vi "PID.vi"(6 "stop":bool, 7 "Angulo Deseado 2":dbl step=100.0, 8 "Reset Counter 2":bool, 9 "Reset Counter":bool, 10 "Angulo Deseado 1":dbl) -> (2 "Pulsos 2":i32, 3 "Pulsos 1":i32)   [LabVIEW 2019]
uses:
  <vilib>/Platform/TimedLoop/XDataNode/timing_clust.ctl
  <vilib>/Platform/TimedLoop/XDataNode/nitl_modes.ctl
  <vilib>/Platform/TimedLoop/XDataNode/wakeup.ctl
  <vilib>/myRIO/Common/Instrument Driver Framework/myRIO v1.0/Encoder/typedefs/Encoder Signal Mode.ctl
  <vilib>/myRIO/Common/Instrument Driver Framework/myRIO v1.0/UART/vis/myRIO v1.0 Close UART.vi
  <vilib>/Utility/error.llb/Error Cluster From Error Code.vi
  <vilib>/myRIO/Common/Instrument Driver Framework/myRIO v1.0/Encoder/vis/myRIO v1.0 Read Encoder.vi
  <vilib>/myRIO/Common/Instrument Driver Framework/myRIO v1.0/PWM/vis/myRIO v1.0 Write PWM.vi
  <vilib>/myRIO/Common/Instrument Driver Framework/myRIO v1.0/DIO/vis/myRIO v1.0 Write DIO.vi
  <vilib>/myRIO/Common/Instrument Driver Framework/Utilities/vis/FPGA Ref Manager.vi
  <vilib>/myRIO/Common/Instrument Driver Framework/myRIO v1.0/myRIO v1.0 Reset FPGA.vi
  <vilib>/myRIO/Common/Instrument Driver Framework/myRIO v1.0/IRQ/vis/myRIO v1.0 IRQ Info FGV.vi
  <vilib>/myRIO/Common/Instrument Driver Framework/myRIO v1.0/IRQ/vis/myRIO v1.0 Timer IRQ Info FGV.vi
  <vilib>/myRIO/Common/Instrument Driver Framework/myRIO v1.0/IRQ/vis/myRIO v1.0 ISR Agent.vi
  <vilib>/myRIO/Instrument Drivers/Utilities/vis/Reset Index.vi
  <vilib>/myRIO/Common/Instrument Driver Framework/myRIO v1.0/Resource Manager/vis/myRIO v1.0 Block Write Resource Manager.vi
  <vilib>/platform/TimedLoop/XDataNode/XDataNode.xnode
  <vilib>/Platform/TimedLoop/XDataNode/XDNodeRunTimeDep.lvlib
  <vilib>/myRIO/Instrument Drivers/Onboard IO/Encoder/Encoder.lvlib
  <vilib>/myRIO/Instrument Drivers/Onboard IO/PWM/PWM.lvlib
  <vilib>/myRIO/Instrument Drivers/Onboard IO/DIO/DIO.lvlib
  <vilib>/myRIO/Instrument Drivers/Utilities/Utilities.lvlib
panel:
  out "Numeric":dbl
  out "Td2":dbl
  out "Ti2":dbl
  out "Kp2":dbl
  out "Td1":dbl
  out "Ti1":dbl
  out "Kp1":dbl
  in  "error 2":dbl
  in  "error":dbl
  out "Waveform Chart":dbl(graph)
  in  "Wc filtro digital 2":dbl
  in  "Wc filtro digital":dbl
  out "Tiempo de muestreo":dbl
  out "?":cluster{dbl, dbl}(graph)
  out "?":cluster{dbl, dbl}(graph)
  out "Angulo Motor 1":dbl
  out "Angulo Motor 2":dbl
  out "Velocidad Motor1":dbl caption="rad/s"
  out "Velocidad Motor2":dbl caption="rad/s"
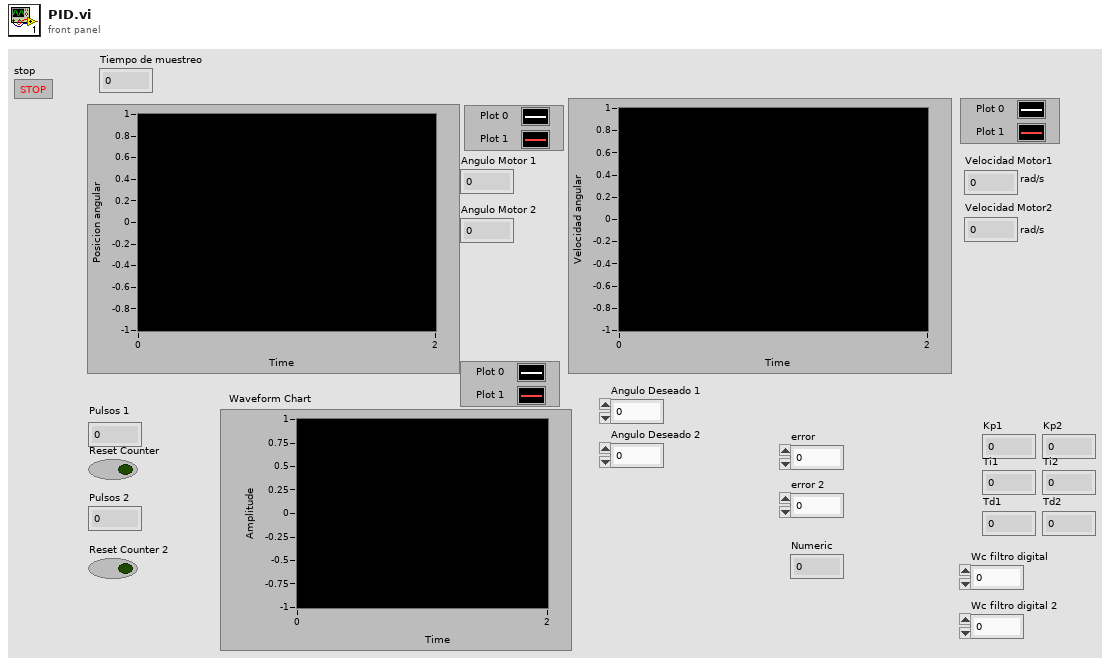
[diagram p1: front panel]
types:
  T1 = typedef "XDNodeRunTimeDep.lvlib/timing_clust.ctl" = cluster{"Expected End [f-1]":u64, "Actual End [f-1]":u64, "Finished Late? [f-1]":bool, "Expected End [i-1]":u64, "Actual End [i-1]":u64, "Finished Late? [i-1]":bool, "Expected Start [i]":u64, "Actual Start [i]":u64, "Expected Start [f]":u64, "Actual Start [f]":u64, "Source Name":string, "Structure Name":string, "Period":i64, "Deadline":i64, "Offset":i64, "Start":i64, "Priority":i32, "Timeout":i32, "Mode":T2, "Wakeup Reason":T3, "Error":errorcluster, "Source Type":string, "Secondary Source Type":string, "Global End Time":u64, "Global Start Time":u64, "Frame Duration":u64, "Iteration Duration":u64, "Assigned CPU":i32, "I/O Scan Engine Mode":u32}
  T2 = typedef "XDNodeRunTimeDep.lvlib/nitl_modes.ctl" = enum32{"No Change", "Process missed periods, maintain original phase", "Discard missed periods, maintain original phase", "Process missed periods, ignore original phase", "Discard missed periods, ignore original phase"}
  T3 = typedef "XDNodeRunTimeDep.lvlib/wakeup.ctl" = enum32{"Normal", "Aborted", "Asynchronous wakeup", "Timing source error", "Timed loop error", "Timeout"}
  T4 = typedef "PWM.lvlib/PWM Reference.ctl" = cluster{"myRIO Reference":T5, "PWM Channels Enum":T9, "PWM Configuration":T10}
  T5 = typedef "myRIO Generic Hardware Reference.ctl" = cluster{"myRIO Model":T6, "myRIO Hardware Reference":T7}
  T6 = typedef "Hardware Version Enum.ctl" = enum16{"Unknown", "myRIO-1900", "myRIO-1950", "roboRIO", "NI ELVIS RIO CM", "ELVIS III"}
  T7 = typedef "myRIO v1.0 Reference.ctl" = cluster{"Generic FPGA Reference":T8, "Allow multiple opens":bool}
  T8 = typedef "Generic FPGA Reference.ctl" = refnum<k20>
  T9 = typedef "PWM Channels Enum.ctl" = enum16{"Not Connected", "C/PWM0", "C/PWM1", "A/PWM0", "A/PWM1", "A/PWM2", "A/PWM3", "A/PWM4", "A/PWM5", "A/PWM6", "A/PWM7", "A/PWM8", "A/PWM9", "A/PWM10", "A/PWM11", "A/PWM12", "A/PWM13", "A/PWM14", "A/PWM15", "A/PWM16", "A/PWM17", "A/PWM18", "A/PWM19", "B/PWM0", "B/PWM1", "B/PWM2", "B/PWM3", "B/PWM4", "B/PWM5", "B/PWM6", "B/PWM7", "B/PWM8", "B/PWM9", "B/PWM10", "B/PWM11", "B/PWM12", "B/PWM13", "B/PWM14", "B/PWM15", "B/PWM16", "B/PWM17", "B/PWM18", "B/PWM19", "PWM/PWM0", "PWM/PWM1", "PWM/PWM2", "PWM/PWM3", "PWM/PWM4", "PWM/PWM5", "PWM/PWM6", "PWM/PWM7", "PWM/PWM8", "PWM/PWM9"}
  T10 = typedef "PWM.lvlib/PWM Configuration.ctl" = cluster{"Frequency":dbl, "Duty Cycle":dbl}
  T11 = typedef "DIO.lvlib/DIO Reference.ctl" = cluster{"myRIO Reference":T5, "DIO Channels List":T12}
  T12 = typedef "DIO Channels List.ctl" = T13[]
  T13 = typedef "DIO Channels Enum.ctl" = enum16{"Not Connected", "C/DIO0", "C/DIO1", "C/DIO2", "C/DIO3", "C/DIO4", "C/DIO5", "C/DIO6", "C/DIO7", "A/DIO0", "A/DIO1", "A/DIO2", "A/DIO3", "A/DIO4", "A/DIO5", "A/DIO6", "A/DIO7", "A/DIO8", "A/DIO9", "A/DIO10", "A/DIO11", "A/DIO12", "A/DIO13", "A/DIO14", "A/DIO15", "A/DIO16", "A/DIO17", "A/DIO18", "A/DIO19", "B/DIO0", "B/DIO1", "B/DIO2", "B/DIO3", "B/DIO4", "B/DIO5", "B/DIO6", "B/DIO7", "B/DIO8", "B/DIO9", "B/DIO10", "B/DIO11", "B/DIO12", "B/DIO13", "B/DIO14", "B/DIO15", "B/DIO16", "B/DIO17", "B/DIO18", "B/DIO19", "LED0", "LED1", "LED2", "LED3", "Button0", "DIO/DIO0", "DIO/DIO1", "DIO/DIO2", "DIO/DIO3", "DIO/DIO4", "DIO/DIO5", "DIO/DIO6", "DIO/DIO7", "DIO/DIO8", "DIO/DIO9", "SPI/CS0", "SPI/CS1", "SPI/CS2", "SPI/CS3", "LED RADIO (Green)", "LED RADIO (Red)", "LED COMM (Green)", "LED COMM (Red)", "LED MODE (Green)", "LED MODE (Red)"}
  T14 = typedef "Encoder Signal Mode.ctl" = enum16{"Quadrature phase signal", "Step and direction signal"}
  T15 = typedef "Encoder.lvlib/Encoder Reference.ctl" = cluster{"myRIO Reference":T5, "Encoder Channels Enum":T16}
  T16 = typedef "Encoder Channels Enum.ctl" = enum16{"Not Connected", "C/ENC0", "C/ENC1", "A/ENC", "A/ENC0", "A/ENC1", "A/ENC2", "A/ENC3", "A/ENC4", "A/ENC5", "A/ENC6", "A/ENC7", "A/ENC8", "A/ENC9", "B/ENC", "B/ENC0", "B/ENC1", "B/ENC2", "B/ENC3", "B/ENC4", "B/ENC5", "B/ENC6", "B/ENC7", "B/ENC8", "B/ENC9", "DIO/ENC0", "DIO/ENC1", "DIO/ENC2", "DIO/ENC3", "DIO/ENC4"}
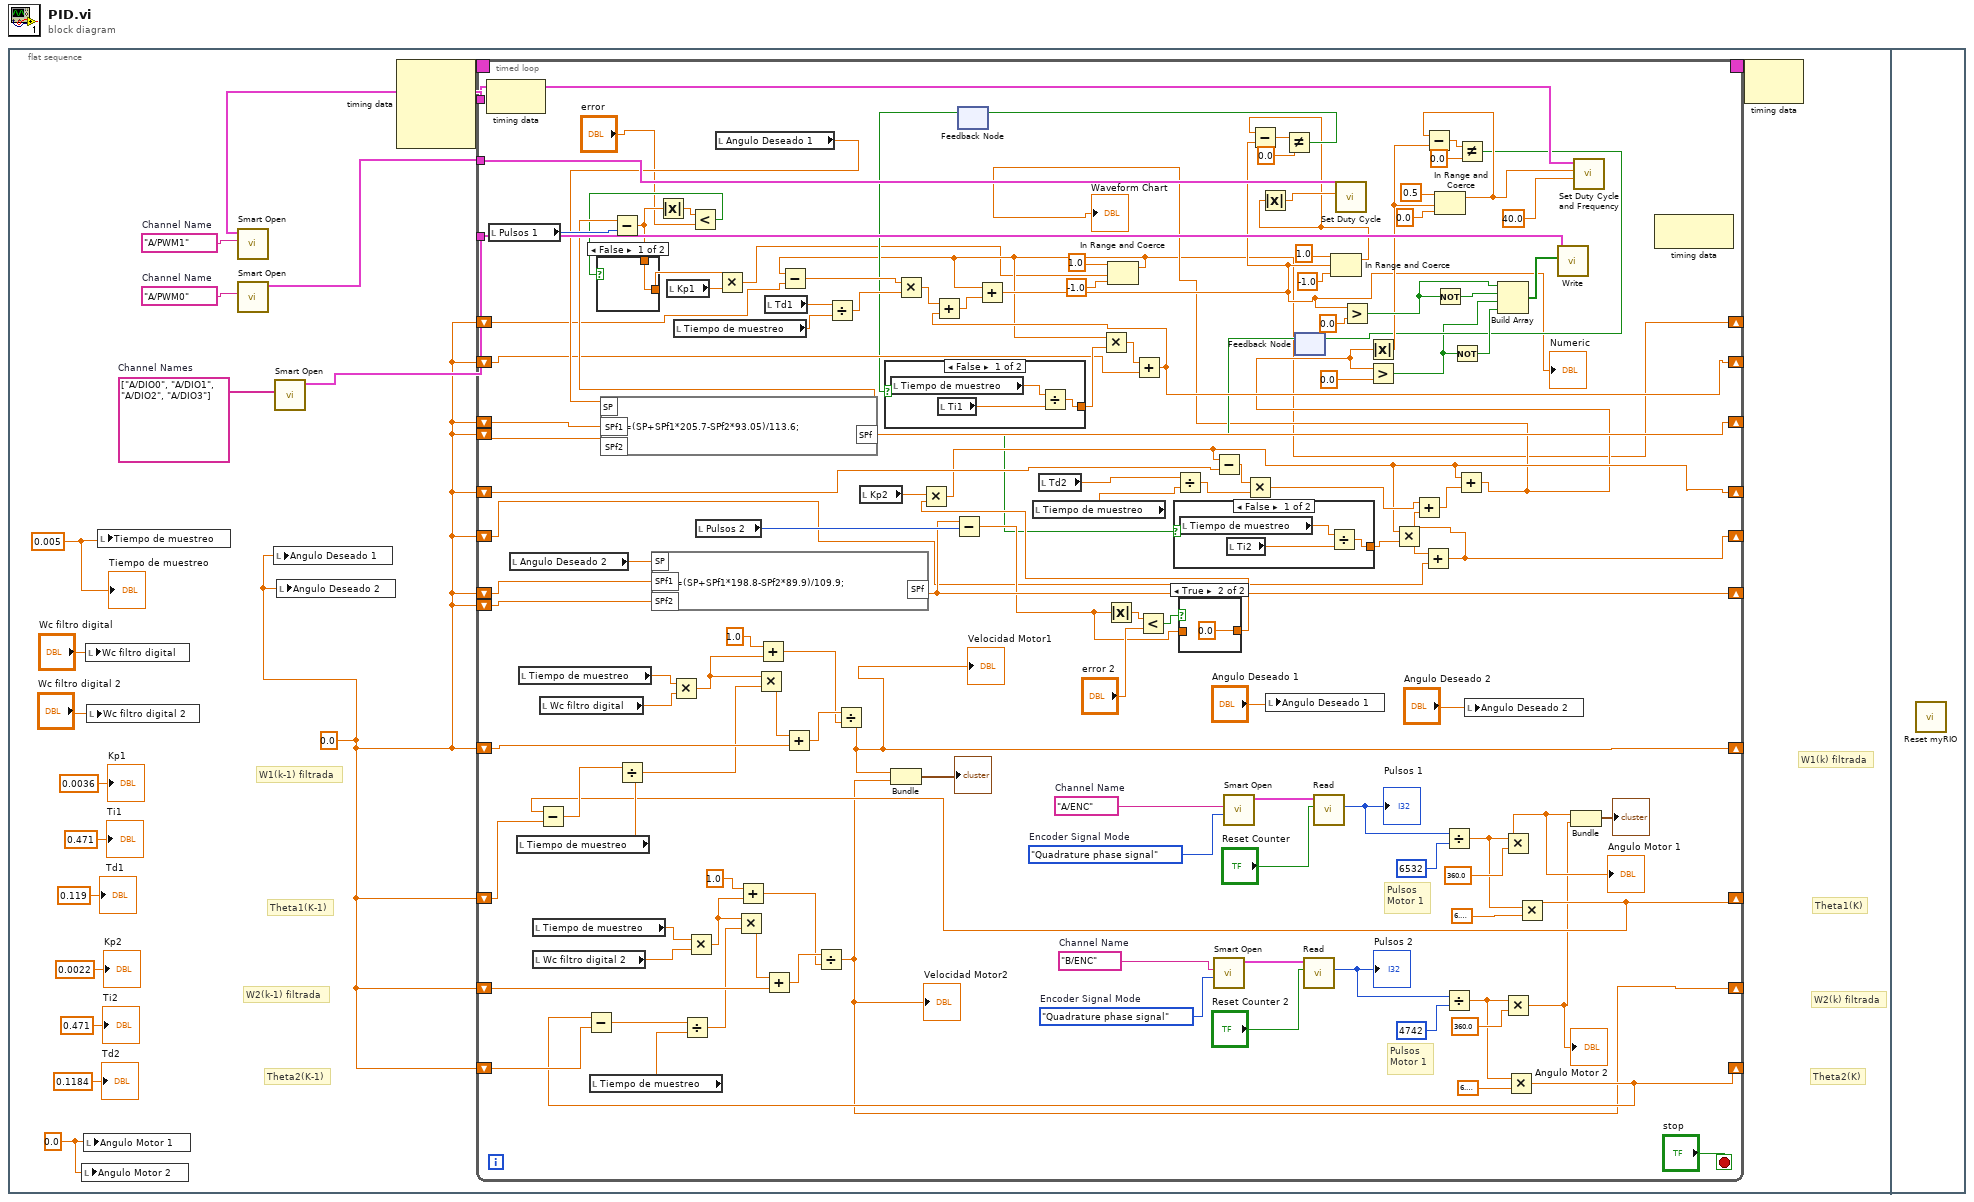
[diagram p0: block diagram]
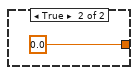
[diagram p2: hidden frame]
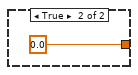
[diagram p3: hidden frame]
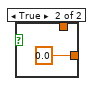
[diagram p5: hidden frame]
diagram:
  n1 = flat-sequence {
    frame #0 {
      w9 = tag "A/PWM1"  # Channel Name
      w1 = 0.0
      w10 = 0.0 ("Angulo Motor 1")
      w12 = tag[] ["A/DIO0", "A/DIO1", "A/DIO2", "A/DIO3"]  # Channel Names
      w15 = 0.005 ("Tiempo de muestreo")
      w16 = tag "A/PWM0"  # Channel Name
      # "W1(k-1) filtrada"
      # "W1(k) filtrada"
      # "Theta1(K-1)"
      # "Theta2(K-1)"
      # "W2(k-1) filtrada"
      # "Theta1(K)"
      # "Theta2(K)"
      # "W2(k) filtrada"
      n2 = local write "Angulo Motor 2"(w10) -> ()
      n3 = local write "Angulo Motor 1"(w10) -> ()
      n4 = local write "Wc filtro digital"("Wc filtro digital") -> ()
      n5 = local write "Wc filtro digital 2"("Wc filtro digital 2") -> ()
      n6 = local write "Tiempo de muestreo"(w15) -> ()
      n7 = call <vilib>:"Smart Open.vi"("Channel Name"=w9) -> ("PWM Ref Out"=w8:T4)  [unwired: 9 in, 1 out]
      n8 = call <vilib>:"Smart Open.vi"("Channel Name"=w16) -> ("PWM Ref Out"=w17:T4)  [unwired: 9 in, 1 out]
      n9 = local write "Angulo Deseado 1"(w1) -> ()
      n10 = call <vilib>:"Smart Open.vi"("Channel Names"=w12) -> ("DIO Ref Out"=w11:T11)  [unwired: 9 in, 1 out]
      n11 = local write "Angulo Deseado 2"(w1) -> ()
      n12 = node-c288() -> (w19:T1)  [unwired: 4 in]
      n13 = timed-loop {
        timing: w19 -> [_]
        timing-out: [_] -> w18
        shift-right: [w129] -> _
        shift-left: w1 -> [w130]
        shift-right: [w104] -> _
        shift-left: w1 -> [w131]
        tunnel: w17 -> [w123]
        shift-right: [w100] -> _
        shift-left: w1 -> [w118]
        shift-right: [w99] -> _
        shift-left: w1 -> [w107]
        tunnel: w11 -> [w105]
        tunnel: w8 -> [w69]
        shift-right: [w40] -> _
        shift-left: w1 -> [w41]
        shift-right: [w37] -> _
        shift-left: w1 -> [w45]
        shift-right: [w83] -> _
        shift-left: w1 -> [w85]
        shift-left: w1 -> [w84]
        shift-right: [w78] -> _
        shift-left: w1 -> [w81]
        shift-left: w1 -> [w80]
        shift-right: [w22] -> _
        shift-left: w1 -> [w62]
        shift-right: [w58] -> _
        shift-left: w1 -> [w59]
        stop <- "stop" stop-if-true
        w145 = Encoder_Signal_Mode."Quadrature phase signal"  # Encoder Signal Mode
        w146 = tag "B/ENC"  # Channel Name
        w149 = Encoder_Signal_Mode."Quadrature phase signal"  # Encoder Signal Mode
        w150 = tag "A/ENC"  # Channel Name
        # "Pulsos\nMotor 1"
        # "Pulsos\nMotor 1"
        n14 = node-c288() -> ()  [unwired: 1 in, 1 out]
        n15 = local read "Pulsos 1"() -> (w79:i32)
        n16 = local read "Angulo Deseado 2"() -> (w86:dbl)
        n17 = local read "Tiempo de muestreo"() -> (w125:dbl)
        n18 = local read "Tiempo de muestreo"() -> (w121:dbl)
        n19 = local read "Tiempo de muestreo"() -> (w120:dbl)
        n20 = local read "Wc filtro digital 2"() -> (w119:dbl)
        n21 = local read "Wc filtro digital"() -> (w122:dbl)
        n22 = local read "Tiempo de muestreo"() -> (w124:dbl)
        n23 = formula code="SPf=(SP+SPf1*198.8-SPf2*89.9)/109.9;"("SPf1"=w85, "SPf2"=w84, "SP"=w86) -> ("SPf"=w83:dbl)
        n24 = local read "Kp1"() -> (w68:dbl)
        n25 = Multiply(x=w121, y=w122) -> (x*y=w108:dbl)
        n26 = local read "Tiempo de muestreo"() -> (w66:dbl)
        n27 = Multiply(x=w120, y=w119) -> (x*y=w115:dbl)
        n28 = local read "Pulsos 2"() -> (w87:i32)
        n29 = local read "Angulo Deseado 1"() -> (w73:dbl)
        n30 = formula code="SPf=(SP+SPf1*205.7-SPf2*93.05)/113.6;"("SPf1"=w81, "SPf2"=w80, "SP"=w73) -> ("SPf"=w78:dbl)
        n31 = Subtract(x=w78, y=w79) -> (x-y=w74:dbl)
        n32 = Absolute Value(x=w74) -> (abs(x)=w76:dbl)
        n33 = Less?(x=w76, y="error") -> (x < y?=w75:bool)
        n34 = case shown="False" w75 {
          tunnel: [w161 0.0] -> w67
          tunnel: w74 -> [w161 _]
          frame False {
          }
          frame True {
          }
        }
        n35 = Multiply(x=w67, y=w68) -> (x*y=w21:dbl)
        n36 = Add(x=1.0, y=w115) -> (x+y=w112:dbl)
        n37 = Add(x=1.0, y=w108) -> (x+y=w109:dbl)
        n38 = local read "Td1"() -> (w65:dbl)
        n39 = Divide(x=w65, y=w66) -> (x/y=w64:dbl)
        n40 = local read "Kp2"() -> (w48:dbl)
        n41 = Subtract(x=w83, y=w87) -> (x-y=w47:dbl)
        n42 = feedback #1() -> (w52:bool)  [unwired: 1 in]
        n43 = case shown="False" w52 {
          tunnel: [w155 0.0] -> w61
          frame False {
            n44 = local read "Tiempo de muestreo"() -> (w156:dbl)
            n45 = local read "Ti1"() -> (w157:dbl)
            n46 = Divide(x=w156, y=w157) -> (x/y=w155:dbl)
          }
          frame True {
          }
        }
        n47 = local read "Tiempo de muestreo"() -> (w51:dbl)
        n48 = local read "Td2"() -> (w50:dbl)
        n49 = Absolute Value(x=w47) -> (abs(x)=w71:dbl)
        n50 = In Range and Coerce(upper limit=1.0, x=w21, lower limit=-1.0) -> (coerced(x)=w22:dbl)  [unwired: 1 out]
        n51 = Subtract(x=w22, y=w62) -> (x-y=w63:dbl)
        n52 = Multiply(x=w63, y=w64) -> (x*y=w57:dbl)
        n53 = Multiply(x=w22, y=w61) -> (x*y=w60:dbl)
        n54 = Add(x=w60, y=w59) -> (x+y=w58:dbl)
        n55 = Add(x=w57, y=w58) -> (x+y=w56:dbl)
        n56 = Add(x=w22, y=w56) -> (x+y=w26:dbl)
        "Numeric" <- w26
        n57 = Less?(x=w71, y="error 2") -> (x < y?=w30:bool)
        n58 = Divide(x=w50, y=w51) -> (x/y=w49:dbl)
        n59 = case shown="True" w30 {
          tunnel: [w159 0.0] -> w46
          tunnel: w47 -> [w159 _]
          frame False {
          }
          frame True {
          }
        }
        n60 = Multiply(x=w48, y=w46) -> (x*y=w37:dbl)
        n61 = Subtract(x=w37, y=w45) -> (x-y=w44:dbl)
        n62 = call <vilib>:"Smart Open.vi"("Encoder Signal Mode"=w145, "Channel Name"=w146) -> ("Encoder Ref Out"=w143:T15)  [unwired: 8 in, 1 out]
        n63 = call <vilib>:"Smart Open.vi"("Encoder Signal Mode"=w149, "Channel Name"=w150) -> ("Encoder Ref Out"=w147:T15)  [unwired: 8 in, 1 out]
        n64 = Multiply(x=w44, y=w49) -> (x*y=w39:dbl)
        n65 = local write "Angulo Deseado 1"("Angulo Deseado 1") -> ()
        n66 = feedback #2() -> (w31:bool)  [unwired: 1 in]
        n67 = case shown="False" w31 {
          tunnel: [w151 0.0] -> w43
          frame False {
            n68 = local read "Tiempo de muestreo"() -> (w152:dbl)
            n69 = local read "Ti2"() -> (w153:dbl)
            n70 = Divide(x=w152, y=w153) -> (x/y=w151:dbl)
          }
          frame True {
          }
        }
        n71 = call <vilib>:"Read.vi"("Reset Counter"="Reset Counter 2", "Encoder Ref In"=w143) -> ("Counter Value"=w136:i32)  [unwired: 5 in, 4 out]
        "Pulsos 2" <- w136
        n72 = call <vilib>:"Read.vi"("Reset Counter"="Reset Counter", "Encoder Ref In"=w147) -> ("Counter Value"=w142:i32)  [unwired: 5 in, 4 out]
        "Pulsos 1" <- w142
        n73 = In Range and Coerce(upper limit=1.0, x=w26, lower limit=-1.0) -> (coerced(x)=w27:dbl)  [unwired: 1 out]
        n74 = Subtract(x=w27, y=w26) -> (x-y=w55:dbl)
        n75 = Absolute Value(x=w27) -> (abs(x)=w28:dbl)
        n76 = Not Equal?(x=w55, y=0.0) -> (x != y?=w53:bool)
        n77 = feedback-in #1(w53) -> ()
        n78 = call <vilib>:"Set Duty Cycle.vi"("Duty Cycle"=w28, "PWM Ref In"=w123) -> ()  [unwired: 7 in, 2 out]
        n79 = Greater?(x=w26, y=0.0) -> (0:w82:bool)
        n80 = Multiply(x=w37, y=w43) -> (x*y=w42:dbl)
        n81 = Add(x=w42, y=w41) -> (x+y=w40:dbl)
        n82 = Add(x=w39, y=w40) -> (x+y=w38:dbl)
        n83 = Not(x=w82) -> (.not. x?=w97:bool)
        n84 = Divide(x=w142, y=6532) -> (x/y=w135:dbl)
        n85 = Divide(x=w136, y=4742) -> (x/y=w133:dbl)
        n86 = Add(x=w37, y=w38) -> (x+y=w25:dbl)
        "Waveform Chart" <- w25
        n87 = Absolute Value(x=w25) -> (abs(x)=w36:dbl)
        n88 = Greater?(x=w25, y=0.0) -> (0:w29:bool)
        n89 = In Range and Coerce(upper limit=0.5, x=w36, lower limit=0.0) -> (coerced(x)=w35:dbl)  [unwired: 1 out]
        n90 = Subtract(x=w35, y=w36) -> (x-y=w34:dbl)
        n91 = Not(x=w29) -> (.not. x?=w95:bool)
        n92 = Not Equal?(x=w34, y=0.0) -> (x != y?=w32:bool)
        n93 = feedback-in #2(w32) -> ()
        n94 = local write "Angulo Deseado 2"("Angulo Deseado 2") -> ()
        n95 = Build Array(w82, w97, w29, w95) -> (w101:bool[])
        n96 = Multiply(x=w135, y=360.0) -> (x*y=w103:dbl)
        "Angulo Motor 1" <- w103
        n97 = Multiply(x=w133, y=360.0) -> (x*y=w102:dbl)
        "Angulo Motor 2" <- w102
        n98 = Multiply(x=w133, y=6.283185307179586) -> (x*y=w129:dbl)
        n99 = Subtract(x=w129, y=w130) -> (x-y=w128:dbl)
        n100 = Divide(x=w128, y=w124) -> (x/y=w117:dbl)
        n101 = Multiply(x=w115, y=w117) -> (x*y=w116:dbl)
        n102 = Add(x=w116, y=w118) -> (x+y=w113:dbl)
        n103 = Divide(x=w113, y=w112) -> (x/y=w100:dbl)
        "Velocidad Motor2" <- w100
        n104 = Multiply(x=w135, y=6.283185307179586) -> (x*y=w104:dbl)
        n105 = Subtract(x=w104, y=w131) -> (x-y=w127:dbl)
        n106 = Divide(x=w127, y=w125) -> (x/y=w106:dbl)
        n107 = Multiply(x=w108, y=w106) -> (x*y=w111:dbl)
        n108 = Add(x=w111, y=w107) -> (x+y=w110:dbl)
        n109 = Divide(x=w110, y=w109) -> (x/y=w99:dbl)
        "Velocidad Motor1" <- w99
        n110 = Bundle(w99, w100) -> (→"?":cluster{dbl, dbl})  [unwired: 1 in]
        n111 = call <vilib>:"Write.vi"("Values"=w101, "DIO Ref In"=w105) -> ()  [unwired: 7 in, 2 out]
        n112 = Bundle(w103, w102) -> (→"?":cluster{dbl, dbl})  [unwired: 1 in]
        n113 = call <vilib>:"Set Duty Cycle and Frequency.vi"("Frequency [Hz]"=40.0, "Duty Cycle"=w35, "PWM Ref In"=w69) -> ()  [unwired: 6 in, 2 out]
        n114 = node-c288() -> ()  [unwired: 1 in, 1 out]
      }
      n115 = node-c288(w18) -> ()  [unwired: 1 out]
      "Tiempo de muestreo" <- w15
      "Kp1" <- 0.0036 ("Kp1")
      "Ti1" <- 0.471 ("Ti")
      "Td1" <- 0.119 ("Td")
      "Kp2" <- 0.0022 ("Kp1")
      "Ti2" <- 0.471 ("Ti")
      "Td2" <- 0.1184 ("Td")
    }
    frame #1 {
      n116 = call <vilib>:"Reset myRIO.vi"() -> ()  [unwired: 11 in, 1 out]
    }
  }
